vi "Initialize Attributes.vi"(8 "error in (no error)":errorcluster, 10 "Attribute Data":variant, 11 "CS++GoBangClient in":refnum<class "CS++GoBangClient.lvclass">) -> (0 "error out":errorcluster, 2 "Found?":bool, 3 "CS++GoBangClient out":refnum<class "CS++GoBangClient.lvclass">)   [LabVIEW 2013, in "GoBang.lvlib" / "CS++GoBangClient.lvclass"]
doc: "Initialize object attribute.\n\nUnique resources should be allocated elsewhere!"
uses:
  CS++GoBangClient.lvclass
  Core/Classes/CS++ProcessVariables/SVConnection/SVConnection.lvclass
  Core/Actors/CS++BaseActor/CS++BaseActor.lvclass
  Core/Actors/CS++BaseActor/CS++BaseActor.lvclass/CS++BaseActor.ctl
  Core/Classes/CS++BaseClasses/Factory/CS++Factory.lvclass
  Core/Classes/CS++ProcessVariables/PVConnection/PVConnection.lvclass/PVConnection.ctl
  CS++GoBangClient.lvclass/CS++GoBangClient.ctl
  Core/Classes/CS++ProcessVariables/PVConnection/PVConnection.lvclass
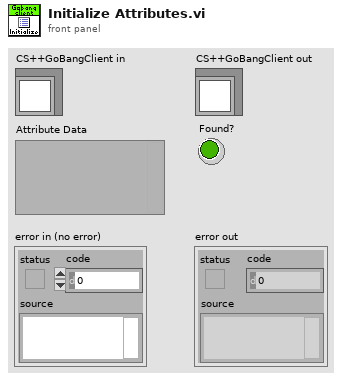
[diagram p1: front panel]
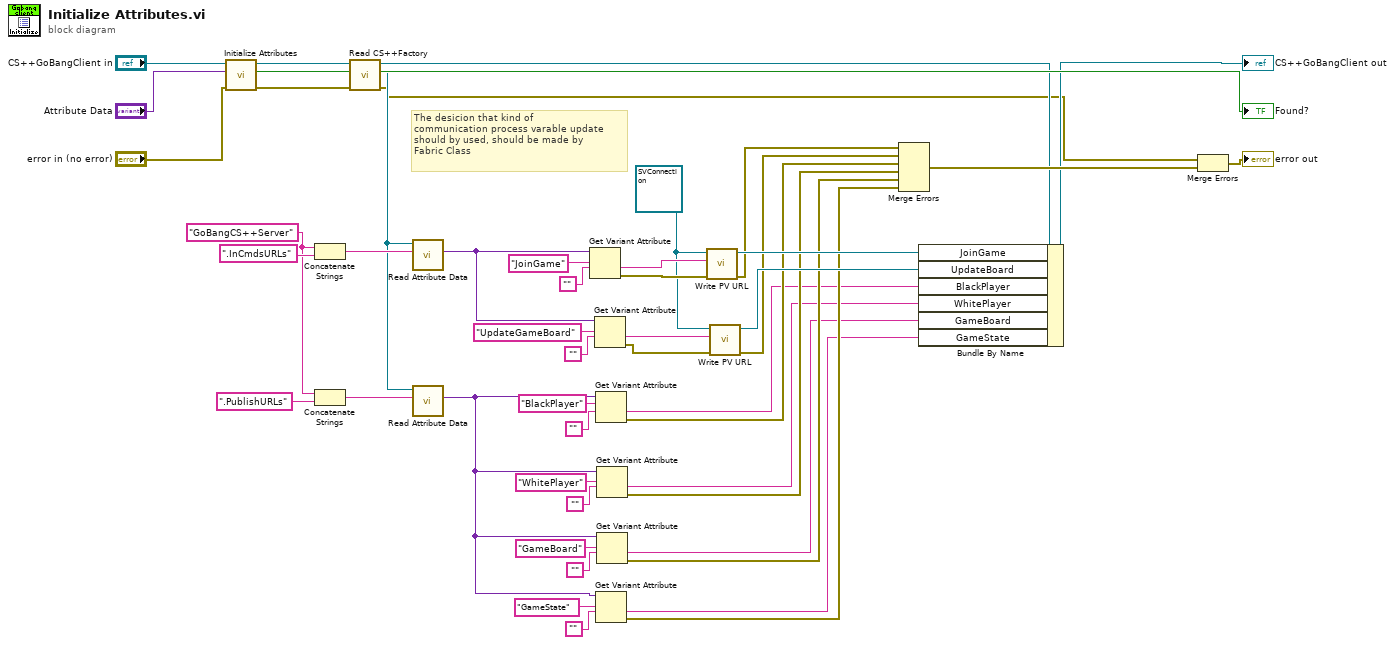
[diagram p0: block diagram]
diagram:
  w19 = "GoBangCS++Server" ("string")
  w20 = refnum<class "SVConnection.lvclass"> refnum ("CS++ProcessVariables.lvlib:SVConnection.lvclass")
  # "The desicion that kind of\ncommunication process varable update \nshould by used, should be made by \nFabric Class"
  n1 = call-parent "Initialize Attributes.vi"("error in (no error)"="error in (no error)", "Attribute Data"="Attribute Data", "CS++BaseActor in"="CS++GoBangClient in") -> ("error out"=w2:errorcluster, "Found?"=→"Found?":bool, "CS++BaseActor out"=w5:refnum<class "CS++GoBangClient.lvclass">)  [unwired: 6 in]
  n2 = Concatenate Strings(w19, ".InCmdsURLs" ("string")) -> (w45:string)
  n3 = Concatenate Strings(w19, ".PublishURLs" ("string")) -> (w26:string)
  n4 = call "Read CS++Factory.vi"("error in (no error)"=w2, "CS++BaseActor in"=w5) -> ("error out"=w1:errorcluster, "CS++Factory"=w23:refnum<class "CS++Factory.lvclass">, "CS++BaseActor out"=w16:refnum<class "CS++GoBangClient.lvclass">)  [unwired: 7 in]
  n5 = call-dynamic "Read Attribute Data.vi"("Object Name"=w45, "CS++Factory in"=w23) -> ("Attribute Data"=w29:variant)  [unwired: 7 in, 2 out]
  n6 = call-dynamic "Read Attribute Data.vi"("Object Name"=w26, "CS++Factory in"=w23) -> ("Attribute Data"=w12:variant)  [unwired: 7 in, 2 out]
  n7 = Get Variant Attribute(Variant=w29, name="JoinGame", default value (empty Variant)="") -> (value=w42:string, error out=w41:errorcluster)  [unwired: 1 in, 2 out]
  n8 = Get Variant Attribute(Variant=w29, name="UpdateGameBoard", default value (empty Variant)="") -> (value=w36:string, error out=w37:errorcluster)  [unwired: 1 in, 2 out]
  n9 = Get Variant Attribute(Variant=w12, name="BlackPlayer", default value (empty Variant)="") -> (value=w10:string, error out=w34:errorcluster)  [unwired: 1 in, 2 out]
  n10 = Get Variant Attribute(Variant=w12, name="GameState", default value (empty Variant)="") -> (value=w7:string, error out=w11:errorcluster)  [unwired: 1 in, 2 out]
  n11 = Get Variant Attribute(Variant=w12, name="WhitePlayer", default value (empty Variant)="") -> (value=w9:string, error out=w30:errorcluster)  [unwired: 1 in, 2 out]
  n12 = Get Variant Attribute(Variant=w12, name="GameBoard", default value (empty Variant)="") -> (value=w8:string, error out=w21:errorcluster)  [unwired: 1 in, 2 out]
  n13 = call "Write PV URL.vi"("error in (no error)"=w41, "PV URL"=w42, "PVConnection in"=w20) -> ("error out"=w28:errorcluster, "PVConnection out"=w40:refnum<class "SVConnection.lvclass">)  [unwired: 7 in]
  n14 = call "Write PV URL.vi"("error in (no error)"=w37, "PV URL"=w36, "PVConnection in"=w20) -> ("error out"=w27:errorcluster, "PVConnection out"=w35:refnum<class "SVConnection.lvclass">)  [unwired: 7 in]
  n15 = Merge Errors(w28, w27, w34, w30, w21, w11) -> (w17:errorcluster)
  n16 = Bundle By Name(cluster=w16, "JoinGame"=w40, "UpdateBoard"=w35, "BlackPlayer"=w10, "WhitePlayer"=w9, "GameBoard"=w8, "GameState"=w7) -> (→"CS++GoBangClient out":refnum<class "CS++GoBangClient.lvclass">)
  n17 = Merge Errors(w1, w17) -> (→"error out":errorcluster)
